vi "enable_Config_subvi.vi"(8 "error in (no error)":errorcluster, 9 "Aardvark Handle":i32 min=0, 10 "Num Bytes to Fetch (64) in":u8=64 min=1, 11 "Address (0x50) in":u16=80 max=1023 format="%.0x") -> (0 "error out":errorcluster, 3 "Data Written":bool)   [LabVIEW 2014]
uses:
  aardvark.dll
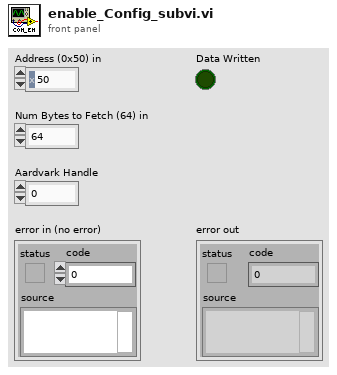
[diagram p1: front panel]
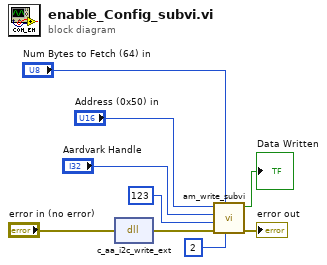
[diagram p0: block diagram]
diagram:
  n1 = dll-call lib="aardvark.dll" fn="c_aa_i2c_write_ext"(error in="error in (no error)") -> (error out=w2:errorcluster)  [unwired: 3 in, 1 out]
  n2 = call "am_write_subvi.vi"("Data to Write"=u8 2, "Num Bytes to Fetch (64)"="Num Bytes to Fetch (64) in", "error in (no error)"=w2, "Memory ADD"=u8 123, "Aardvark Handle in"="Aardvark Handle", "Address (0x50) in"="Address (0x50) in") -> ("error out"=→"error out":errorcluster, "Data Written"=→"Data Written":bool)  [unwired: 4 in]
